vi "img test8(track 2).vi"() -> ()   [LabVIEW 2013]
uses:
  <vilib>/vision/NI_Vision_Development_Module.lvlib
panel:
  in  "frame jump":i32=3
  in  "milliseconds to wait":u32=200
  in  "start":i32
  out "Image 5":T1(plugin-control)
  out "Image 3":T1(plugin-control)
  in  "Range":cluster{"Lower value":sgl, "Upper value":sgl}={"Lower value"=30.0, "Upper value"=90.0} {"Upper value" format="%.2f"; "Lower value" format="%.2f"}
  out "Image 2":T1(plugin-control)
  in  "AVI Path":path=path "C:/Users/Kokum Weeratunga/Desktop/img processing/ChongWei vs LinDan (japan open 2010).avi"
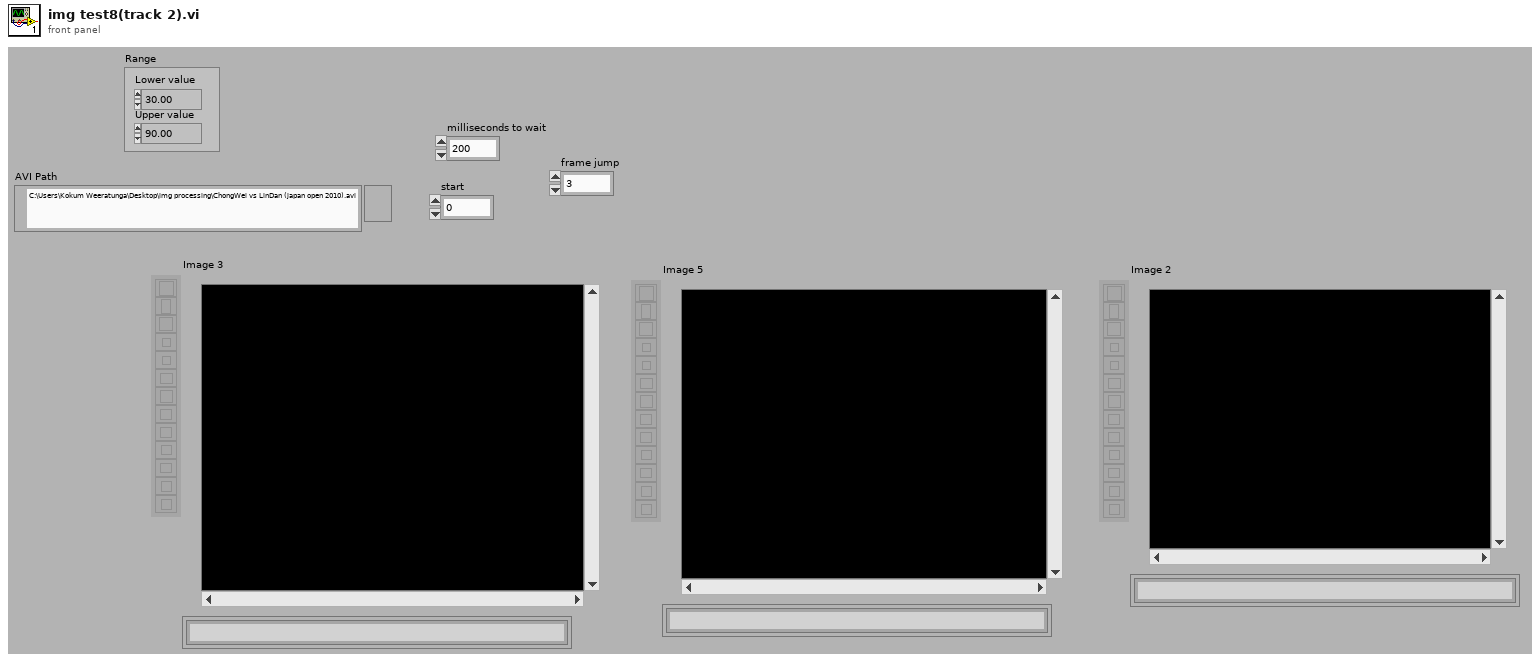
[diagram p1: front panel]
types:
  T1 = typedef "IMAQ Image.ctl" = refnum<image>
  T2 = typedef "Image Type" = u32
  T3 = typedef "AviRefnum.ctl" = refnum<k1>
  T4 = enum32{"AutoM", "Close", "Dilate", "Erode", "Gradient", "Gradient out", "Gradient in", "Hit miss", "Open", "PClose", "POpen", "Thick", "Thin"}
  T5 = enum32{"AutoM", "Close", "Dilate", "Erode", "Gradient", "Gradient in", "Gradient out", "HitMiss", "Open", "PClose", "POpen", "Thick", "Thin"}
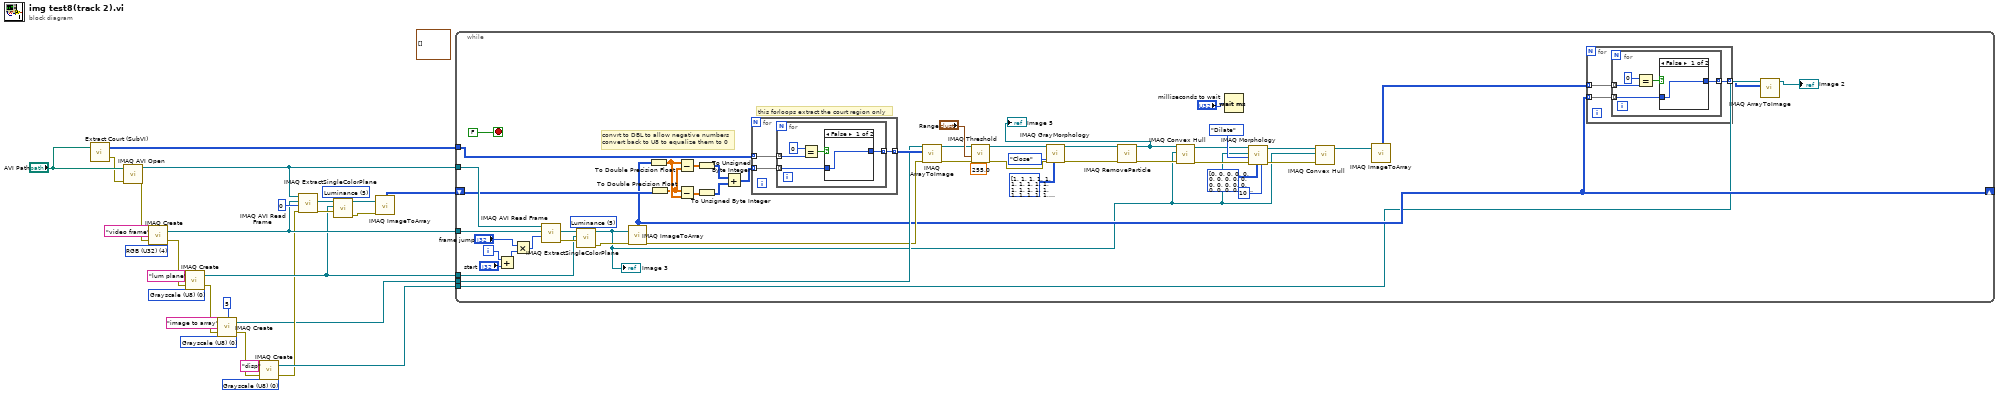
[diagram p0: block diagram]
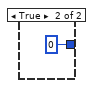
[diagram p2: hidden frame]
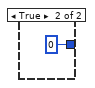
[diagram p3: hidden frame]
diagram:
  (unwired) cluster{"Numeric":dbl, "Numeric":dbl}[] []
  w12 = T2 0 items=["Grayscale (U8)", "Grayscale (I16)", "Grayscale (SGL)", "Complex (CSG)", "RGB (U32)", "HSL (U32)", "RGB (U64)", "Grayscale (U16)"] ("Image Type")
  w20 = 5 items=["Red", "Green", "Blue", "Hue", "Saturation", "Luminance", "Value", "Intensity"] ("Color Plane")
  w22 = T2 0 items=["Grayscale (U8)", "Grayscale (I16)", "Grayscale (SGL)", "Complex (CSG)", "RGB (U32)", "HSL (U32)", "RGB (U64)", "Grayscale (U16)"] ("Image Type")
  w26 = T2 0 items=["Grayscale (U8)", "Grayscale (I16)", "Grayscale (SGL)", "Complex (CSG)", "RGB (U32)", "HSL (U32)", "RGB (U64)", "Grayscale (U16)"] ("Image Type")
  w24 = T2 4 items=["Grayscale (U8)", "Grayscale (I16)", "Grayscale (SGL)", "Complex (CSG)", "RGB (U32)", "HSL (U32)", "RGB (U64)", "Grayscale (U16)"] ("Image Type")
  n1 = call "Extract Court (SubVI).vi"("AVI Path"="AVI Path") -> ("error out"=w28:errorcluster, "Court pixels out"=w2:u8[][])  [unwired: 1 in]
  n2 = call "IMAQ AVI Open"("error in (no error)"=w28, "AVI Path"="AVI Path") -> ("error out"=w8:errorcluster, "Avi Refnum"=w18:T3)  [unwired: 8 in]
  n3 = call "IMAQ Create"("Image Name"="video frame", "Image Type"=w24, "error in (no error)"=w8) -> ("New Image"=w16:T1, "error out"=w7:errorcluster)  [unwired: 2 in]
  n4 = call "IMAQ Create"("Image Name"="lum plane", "Image Type"=w26, "error in (no error)"=w7) -> ("New Image"=w15:T1, "error out"=w6:errorcluster)  [unwired: 2 in]
  n5 = call "IMAQ Create"("Border Size"=5, "Image Name"="image to array", "Image Type"=w22, "error in (no error)"=w6) -> ("New Image"=w1:T1, "error out"=w5:errorcluster)  [unwired: 1 in]
  n6 = call "IMAQ Create"("Image Name"="disp", "Image Type"=w12, "error in (no error)"=w5) -> ("New Image"=w10:T1, "error out"=w4:errorcluster)  [unwired: 2 in]
  n7 = call "IMAQ AVI Read Frame"("error in (no error)"=w4, "Frame Number"=u32 0, "Image"=w16, "Avi Refnum"=w18) -> ("error out"=w19:errorcluster, "Image Out"=w21:T1)  [unwired: 4 in, 2 out]
  n8 = call "IMAQ ExtractSingleColorPlane"("Color Plane"=w20, "error in (no error)"=w19, "Image Dst"=w15, "Image Src"=w21) -> ("error out"=w9:errorcluster, "Image Dst Out"=w13:T1)  [unwired: 6 in]
  n9 = call "IMAQ ImageToArray"("error in (no error)"=w9, "Image"=w13) -> ("Image Pixels (U8)"=w14:u8[][])  [unwired: 2 in, 4 out]
  n10 = while {
    tunnel: w18 -> [w79]
    tunnel: w16 -> [w40]
    tunnel: w2 -> [w78]
    tunnel: w15 -> [w42]
    tunnel: w1 -> [w71]
    shift-right: [w38] -> _
    shift-left: w14 -> [w70]
    tunnel: w10 -> [w36]
    i -> [w63]
    stop <- FALSE stop-if-true
    w80 = 5 items=["Red", "Green", "Blue", "Hue", "Saturation", "Luminance", "Value", "Intensity"] ("Color Plane")
    # "convrt to DBL to allow negative numbers\nconvert back to U8 to equalize them to 0"
    # "this forloops extract the court region only"
    n11 = Add(x=w63, y="start") -> (x+y=w62:i32)
    n12 = Multiply(x="frame jump", y=w62) -> (x*y=w75:i32)
    n13 = call "IMAQ AVI Read Frame"("Frame Number"=w75, "Image"=w40, "Avi Refnum"=w79) -> ("error out"=w81:errorcluster, "Image Out"=w41:T1)  [unwired: 5 in, 2 out]
    n14 = call "IMAQ ExtractSingleColorPlane"("Color Plane"=w80, "error in (no error)"=w81, "Image Dst"=w42, "Image Src"=w41) -> ("error out"=w56:errorcluster, "Image Dst Out"=w31:T1)  [unwired: 6 in]
    "Image 3" <- w31
    n15 = call "IMAQ ImageToArray"("error in (no error)"=w56, "Image"=w31) -> ("error out"=w55:errorcluster, "Image Pixels (U8)"=w38:u8[][])  [unwired: 2 in, 3 out]
    n16 = To Double Precision Float(number=w38) -> (double precision float=w60:dbl[][])
    n17 = To Double Precision Float(number=w70) -> (double precision float=w59:dbl[][])
    n18 = Subtract(x=w60, y=w59) -> (x-y=w58:dbl[][])
    n19 = Subtract(x=w59, y=w60) -> (x-y=w57:dbl[][])
    n20 = To Unsigned Byte Integer(number=w58) -> (unsigned 8bit integer=w69:u8[][])
    n21 = To Unsigned Byte Integer(number=w57) -> (unsigned 8bit integer=w68:u8[][])
    n22 = Add(x=w69, y=w68) -> (x+y=w67:u8[][])
    n23 = for {
      tunnel: w78 -> [w94] mode=indexing
      tunnel: [w93] -> w76 mode=indexing
      tunnel: w67 -> [w92] mode=indexing
      n24 = for {
        tunnel: w94 -> [w99] mode=indexing
        tunnel: [w96] -> w93 mode=indexing
        tunnel: w92 -> [w95] mode=indexing
        n25 = Equal?(x=u8 0, y=w99) -> (x = y?=w97:bool)
        n26 = case shown="False" w97 {
          tunnel: [w100 u8 0 ("x")] -> w96
          tunnel: w95 -> [w100 _]
          frame False {
          }
          frame True {
          }
        }
      }
    }
    n27 = call "IMAQ ArrayToImage"("error in (no error)"=w55, "Image Pixels (U8)"=w76, "Image"=w71) -> ("error out"=w54:errorcluster, "Image Out"=w43:T1)  [unwired: 7 in]
    n28 = call "IMAQ Threshold"("Replace Value"=sgl 255.0, "error in (no error)"=w54, "Range"="Range", "Image Src"=w43) -> ("error out"=w53:errorcluster, "Image Dst Out"=w66:T1)  [unwired: 6 in]
    n29 = call "IMAQ GrayMorphology"("Structuring Element"=i32[][] [[1, 1, 1, 1, 1, 1, 1, 1, 1], [1, 1, 1, 1, 1, 1, 1, 1, 1], [1, 1, 1, 1, 1, 1, 1, 1, 1], [1, 1, 1, 1, 1, 1, 1, 1, 1], [1, 1, 1, 1, 1, 1, 1, 1, 1], [1, 1, 1, 1, 1, 1, 1, 1, 1], [1, 1, 1, 1, 1, 1, 1, 1, 1], [1, 1, 1, 1, 1, 1, 1, 1, 1], [1, 1, 1, 1, 1, 1, 1, 1, 1]], "error in (no error)"=w53, "Operation"=T5."Close", "Image Src"=w66) -> ("error out"=w52:errorcluster, "Image Dst Out"=w33:T1)  [unwired: 6 in]
    n30 = call "IMAQ RemoveParticle"("error in (no error)"=w52, "Image Src"=w33) -> ("error out"=w51:errorcluster, "Image Dst Out"=w30:T1)  [unwired: 8 in]
    "Image 5" <- w30
    n31 = call "IMAQ Convex Hull"("error in (no error)"=w51, "Image Dst"=w31, "Image Src"=w30) -> ("error out"=w47:errorcluster, "Image Dst Out"=w32:T1)  [unwired: 7 in]
    n32 = Wait (ms)(milliseconds to wait="milliseconds to wait") -> ()  [unwired: 1 out]
    n33 = call "IMAQ Morphology"("Number of iterations (1)"=10, "Structuring Element"=i32[][] [[0, 0, 0, 0, 0, 0, 0], [0, 0, 0, 0, 0, 0, 0], [0, 0, 0, 0, 0, 0, 0], [0, 0, 0, 0, 0, 0, 0], [0, 0, 1, 1, 1, 0, 0], [0, 0, 0, 1, 0, 0, 0], [0, 0, 0, 1, 0, 0, 0]], "error in (no error)"=w47, "Operation"=T4."Dilate", "Image Dst"=w31, "Image Src"=w32) -> ("error out"=w44:errorcluster, "Image Dst Out"=w45:T1)  [unwired: 4 in]
    n34 = call "IMAQ Convex Hull"("error in (no error)"=w44, "Image Dst"=w31, "Image Src"=w45) -> ("Image Dst Out"=w37:T1)  [unwired: 7 in, 1 out]
    n35 = call "IMAQ ImageToArray"("Image"=w37) -> ("Image Pixels (U8)"=w39:u8[][])  [unwired: 3 in, 4 out]
    n36 = for {
      tunnel: w39 -> [w84] mode=indexing
      tunnel: [w83] -> w35 mode=indexing
      tunnel: w38 -> [w82] mode=indexing
      n37 = for {
        tunnel: w84 -> [w89] mode=indexing
        tunnel: [w86] -> w83 mode=indexing
        tunnel: w82 -> [w85] mode=indexing
        n38 = Equal?(x=u8 0, y=w89) -> (x = y?=w87:bool)
        n39 = case shown="False" w87 {
          tunnel: [w90 u8 0 ("x")] -> w86
          tunnel: w85 -> [w90 _]
          frame False {
          }
          frame True {
          }
        }
      }
    }
    n40 = call "IMAQ ArrayToImage"("Image Pixels (U8)"=w35, "Image"=w36) -> ("Image Out"=→"Image 2":T1)  [unwired: 8 in, 1 out]
  }
